vi "RichToFlatniswitch_grpc_ConfigureScanListRequest.vi"(5 "OutputClusterType":T1, 11 "InputCluster":T4) -> (3 "OutputCluster":T1)   [LabVIEW 2021, in "NI Switch_client.lvlib"]
uses:
  NI Switch_client.lvlib
  niswitch_grpc_ConfigureScanListRequest.ctl
  niswitch_grpc_ConfigureScanListRequest_scan_mode_enum/niswitch_grpc_ConfigureScanListRequest_scan_mode_enum.lvclass
  nidevice_grpc_Session.ctl
  niswitch_grpc_ConfigureScanListRequest_Flat.ctl
  nidevice_grpc_Session_Flat.ctl
  niswitch_grpc_ScanMode.ctl
  niswitch_grpc_ConfigureScanListRequest_scan_mode_enum/niswitch_grpc_ConfigureScanListRequest_scan_mode_enum.lvclass/niswitch_grpc_ConfigureScanListRequest_scan_mode_enum.ctl
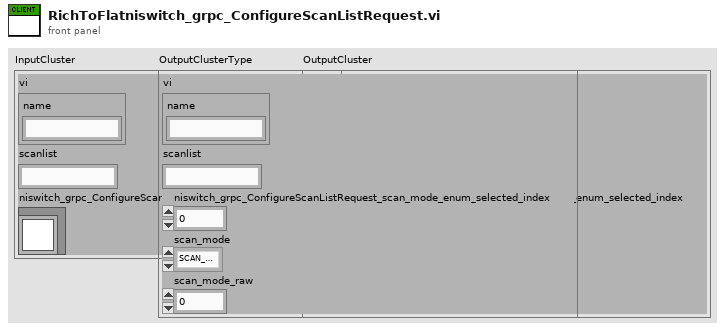
[diagram p1: front panel]
types:
  T1 = typedef "NI Switch_client.lvlib/niswitch_grpc_ConfigureScanListRequest_Flat.ctl" = cluster{"vi":T2, "scanlist":string, "niswitch_grpc_ConfigureScanListRequest_scan_mode_enum_selected_index":i32, "scan_mode":T3, "scan_mode_raw":i32}
  T2 = typedef "NI Switch_client.lvlib/nidevice_grpc_Session_Flat.ctl" = cluster{"name":string}
  T3 = typedef "NI Switch_client.lvlib/niswitch_grpc_ScanMode.ctl" = enum32{"SCAN_MODE_NISWITCH_VAL_NONE", "SCAN_MODE_NISWITCH_VAL_BREAK_BEFORE_MAKE", "SCAN_MODE_NISWITCH_VAL_BREAK_AFTER_MAKE"}
  T4 = typedef "NI Switch_client.lvlib/niswitch_grpc_ConfigureScanListRequest.ctl" = cluster{"vi":T5, "scanlist":string, "niswitch_grpc_ConfigureScanListRequest_scan_mode_enum":refnum<class "niswitch_grpc_ConfigureScanListRequest_scan_mode_enum.lvclass">}
  T5 = typedef "NI Switch_client.lvlib/nidevice_grpc_Session.ctl" = cluster{"name":string}
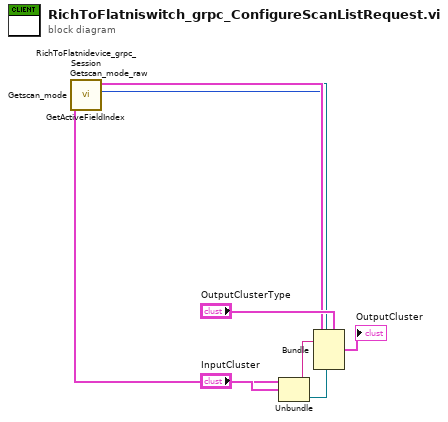
[diagram p0: block diagram]
diagram:
  n1 = Unbundle "Unbundle"("InputCluster") -> ("vi"=w7:T5, "scanlist"=w5:string, "niswitch_grpc_ConfigureScanListRequest_scan_mode_enum"=w4:refnum<class "niswitch_grpc_ConfigureScanListRequest_scan_mode_enum.lvclass">)
  n2 = call "Getscan_mode_raw.vi"("OneOfTemplate in"=w4) -> ("Get_Val"=w1:i32)  [unwired: 8 in, 2 out]
  n3 = call "Getscan_mode.vi"("OneOfTemplate in"=w4) -> ("Get_Val"=w2:T3)  [unwired: 8 in, 2 out]
  n4 = call "GetActiveFieldIndex.vi"("OneOfTemplate in"=w4) -> ("Active Field Index"=w3:i32)  [unwired: 8 in, 2 out]
  n5 = call "RichToFlatnidevice_grpc_Session.vi"("InputCluster"=w7) -> ("OutputCluster"=w6:T2)  [unwired: 10 in]
  n6 = Bundle "Bundle"(cluster="OutputClusterType", "vi"=w6, "scanlist"=w5, "niswitch_grpc_ConfigureScanListRequest_scan_mode_enum_selected_index"=w3, "scan_mode"=w2, "scan_mode_raw"=w1) -> (→"OutputCluster":T1)
